vi "Must Contain Regex.vi"(10 "Must Contain":T1, 11 "Possibles":string[](array[string])) -> (3 "Possibles":string[](array[string]))   [LabVIEW 2025, in "WordleSolver.lvlib"]
uses:
  WordleSolver.lvlib
  Controls/Must Contain.ctl
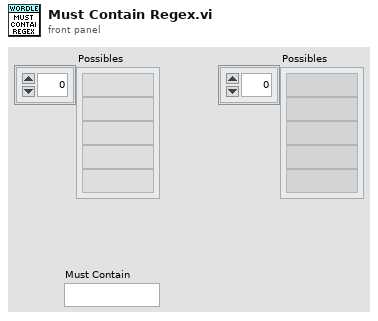
[diagram p1: front panel]
types:
  T1 = typedef "Must Contain.ctl" = string
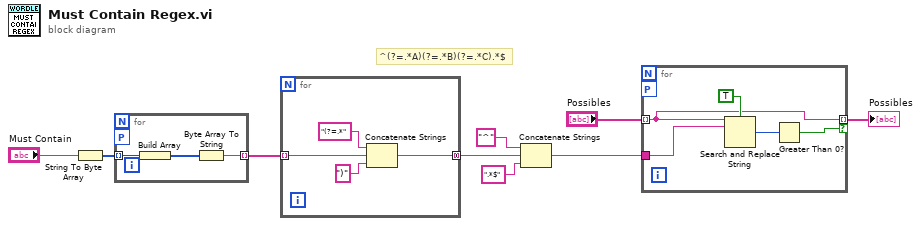
[diagram p0: block diagram]
diagram:
  # "^(?=.*A)(?=.*B)(?=.*C).*$"
  n1 = String To Byte Array(string="Must Contain") -> (unsigned byte array=w8:u8[])
  n2 = for {
    workers-P: _ -> [_]
    tunnel: w8 -> [w12] mode=indexing
    tunnel: [w10] -> w6 mode=indexing
    n3 = Build Array(w12) -> (w11:u8[])
    n4 = Byte Array To String(unsigned byte array=w11) -> (string=w10:string)
  }
  n5 = for {
    tunnel: w6 -> [w14] mode=indexing
    tunnel: [w13] -> w4 mode=concatenating
    n6 = Concatenate Strings("(?=.*" ("string"), w14, ")" ("string")) -> (w13:string)
  }
  n7 = Concatenate Strings("^" ("string"), w4, ".*$" ("string")) -> (w2:string)
  n8 = for {
    tunnel: "Possibles" -> [w18] mode=indexing
    tunnel: w2 -> [w21]
    tunnel: [w18] -> w7 mode=indexing if=w17
    workers-P: _ -> [_]
    n9 = Search and Replace String(case sensitive?=TRUE ("ignore case? (F)"), input string=w18, search string=w21) -> (number of replacements=w19:i32)  [unwired: 5 in, 3 out]
    n10 = Greater Than 0?(x=w19) -> (x > 0?=w17:bool)
  }
  "Possibles" <- w7
